vi "Demo_Main.vi"() -> ()   [LabVIEW 2011]
uses:
  ControlCAN/ControlCAN.llb/DevType.ctl
  ControlCAN/ControlCAN.llb/CAN Channel.ctl
  ControlCAN/ControlCAN.llb/InitFlag.ctl
  ControlCAN/ControlCAN.llb/Mode.ctl
  ControlCAN/ControlCAN.llb/Fliter.ctl
  ControlCAN/ControlCAN.llb/VCI_CAN_OBJ.ctl
  ControlCAN/ControlCAN.llb/VCI_INIT_CONFIG.ctl
  ControlCAN/ControlCAN.llb/Return Val.ctl
  ControlCAN/ControlCAN.lvlib
panel:
  in  "Clear":bool
  out "RecvCnt":u32 caption="接收统计"
  out "SendCnt":u32 caption="发送统计"
  in  "Format":u8(ring) items=["标准帧", "扩展帧"]
  in  "Type":u8(ring) items=["数据帧", "远程帧"]
  in  "Data":string="00 01 02 03 04 05 06 07"
  in  "ID":u32=291 format="0x%x"
  in  "list":i32(listbox)
  in  "Send":bool
  in  "RcvEnable":bool=TRUE
  out "Open":bool
  in  "Fliter":T1=1 items=["接收所有类型"=1, "只接收标准帧"=2, "只接收扩展帧"=3]
  in  "kBaudRate":u8(ring)=15 caption="波特率" items=["5k bps"=1, "10k bps"=2, "20k bps"=3, "40k bps"=4, "50k bps"=5, "80k bps"=6, "100k bps"=7, "125k bps"=8, "200k bps"=9, "250k bps"=10, "400k bps"=11, "500k bps"=12, "666k bps"=13, "800k bps"=14, "1000k bps"=15, "33.33k bps"=16, "66.66k bps"=17, "83.33k bps"=18]
  in  "Mode":T2=2 caption="工作模式" items=["正常工作", "仅侦听模式", "自测模式（环回）"]
  in  "InitFlag":T3=1 caption="保留值" items=["使用界面设置参数"=1]
  in  "AccMask":u32=4294967295 caption="接收屏蔽码" format="%08x"
  in  "AccCode":u32 caption="接收过滤码" format="%08x"
  in  "Close":bool
  in  "Open":bool
  in  "Channel":T4 caption="CAN通道" items=["通道1", "通道2"]
  in  "DevType":T5=4 caption="设备类型" items=["USB-CAN"=3, "USB-CAN2"=4]
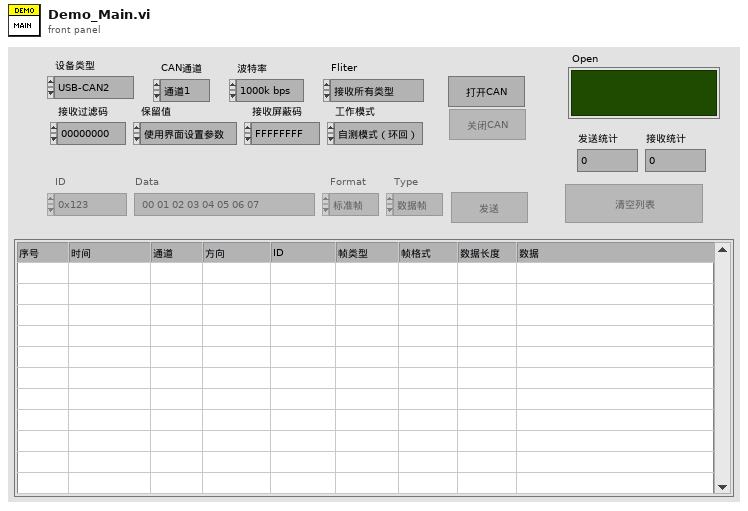
[diagram p1: front panel]
types:
  T1 = typedef "ControlCAN.lvlib/Fliter.ctl" = u8
  T2 = typedef "ControlCAN.lvlib/Mode.ctl" = u8
  T3 = typedef "ControlCAN.lvlib/InitFlag.ctl" = u32
  T4 = typedef "ControlCAN.lvlib/CAN Channel.ctl" = u32
  T5 = typedef "ControlCAN.lvlib/DevType.ctl" = u32
  T6 = typedef "ControlCAN.lvlib/VCI_CAN_OBJ.ctl" = cluster{"ID":u32, "TimeStamp":u32, "TimeFlag":u8, "SendType":u8, "RemoteFlag":u8, "ExternFlag":u8, "DataLen":u8, "Data":u8[], "Reserved":u8[]}
  T7 = cluster{"Type":enum16{"接收", "发送"}, "Channel":T4, "Time":timestamp, "VCI_CAN_OBJ":T6}[]
  T8 = cluster{"Type":enum16{"接收", "发送"}, "Channel":T4, "Time":timestamp, "VCI_CAN_OBJ":T6}
  T9 = typedef "ControlCAN.lvlib/VCI_INIT_CONFIG.ctl" = cluster{"AccCode":u32, "AccMask":u32, "InitFlag":T3, "Fliter":T1, "Timing0":u8, "Timing1":u8, "Mode":T2}
  T10 = cluster{"DevType":T5, "DevIndex":u32, "CanIndex":T4, "VCI_INIT_CONFIG":T9}
  T11 = typedef "ControlCAN.lvlib/Return Val.ctl" = i32
  T12 = enum32{"invalid app kind", "Development System", "Run Time System", "Student Edition", "Embedded LabVIEW", "Evaluation", "Custom"}
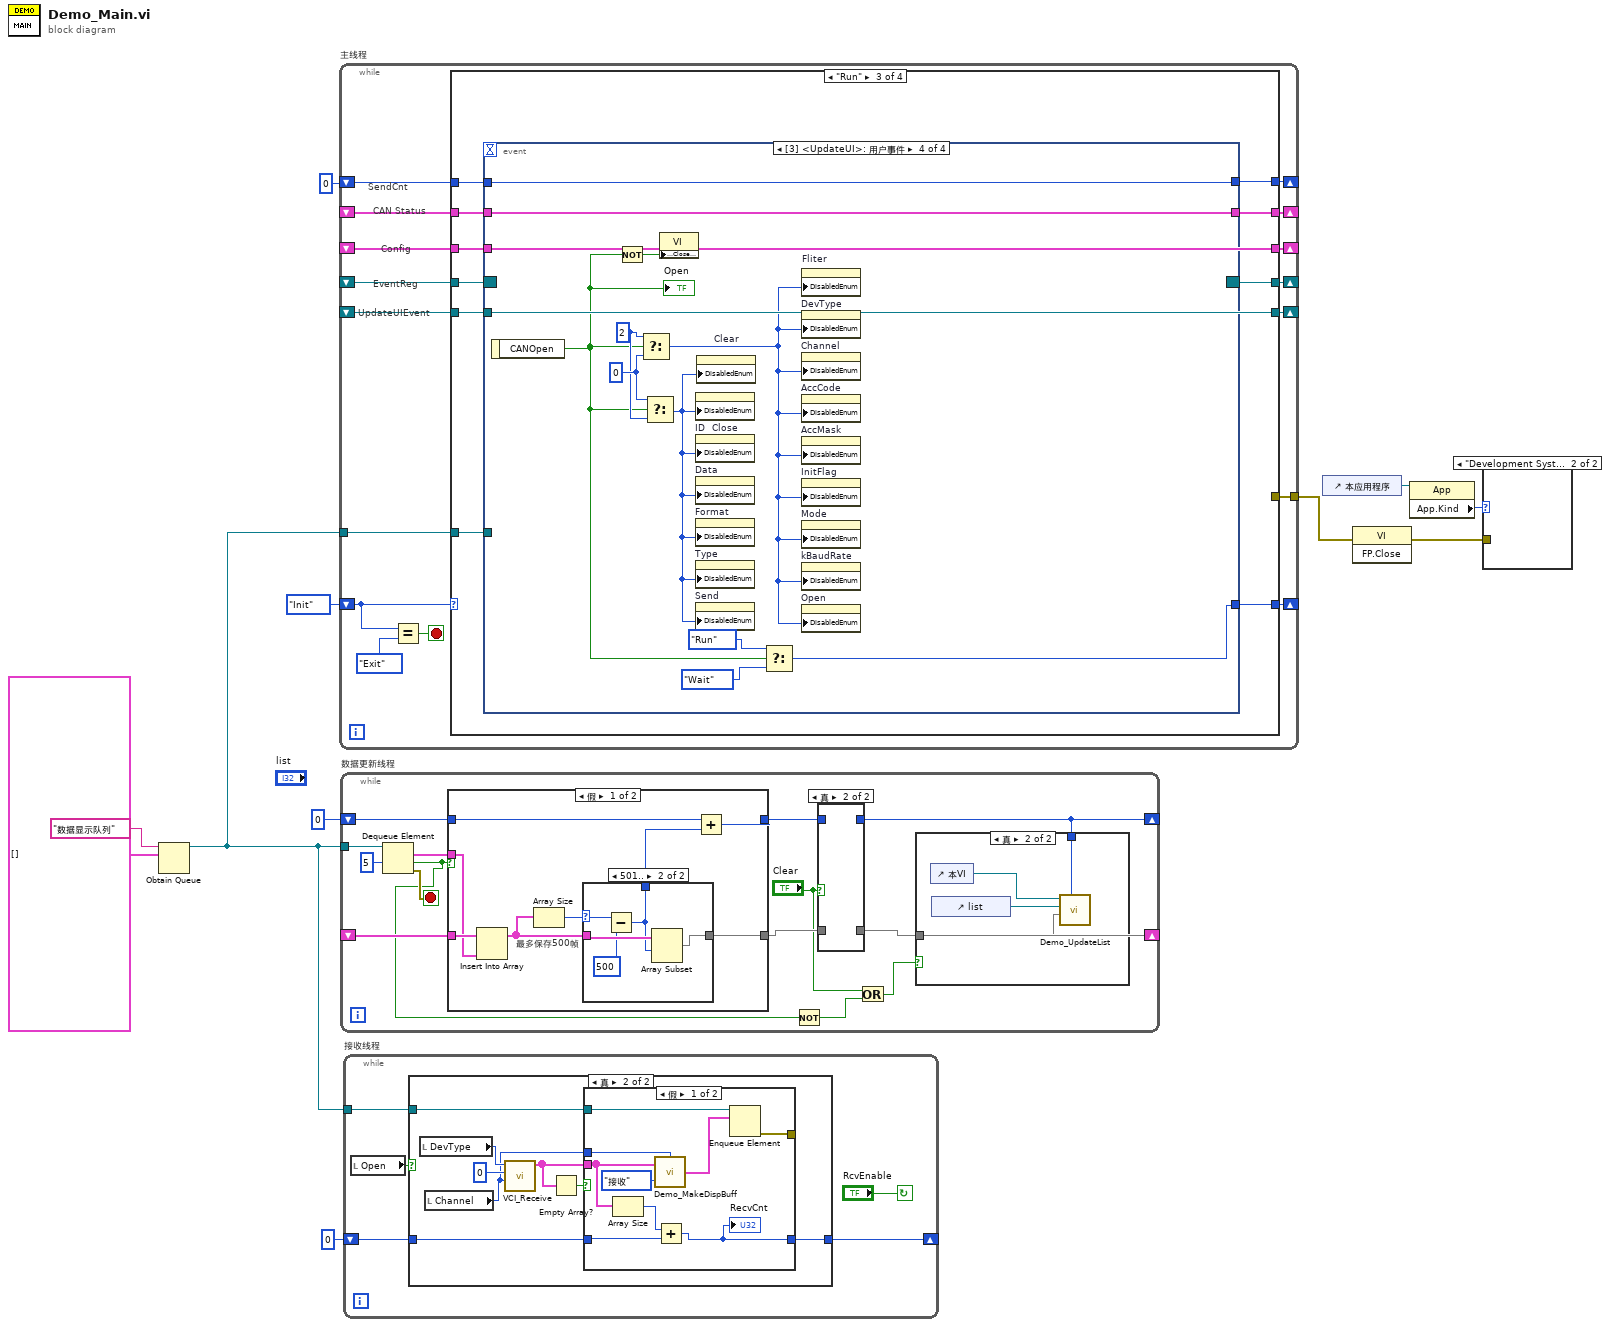
[diagram p0: block diagram]
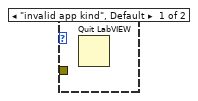
[diagram p2: hidden frame]
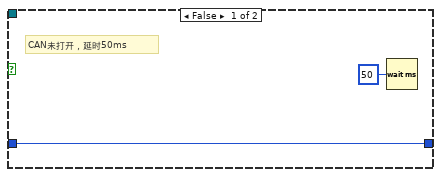
[diagram p7: hidden frame]
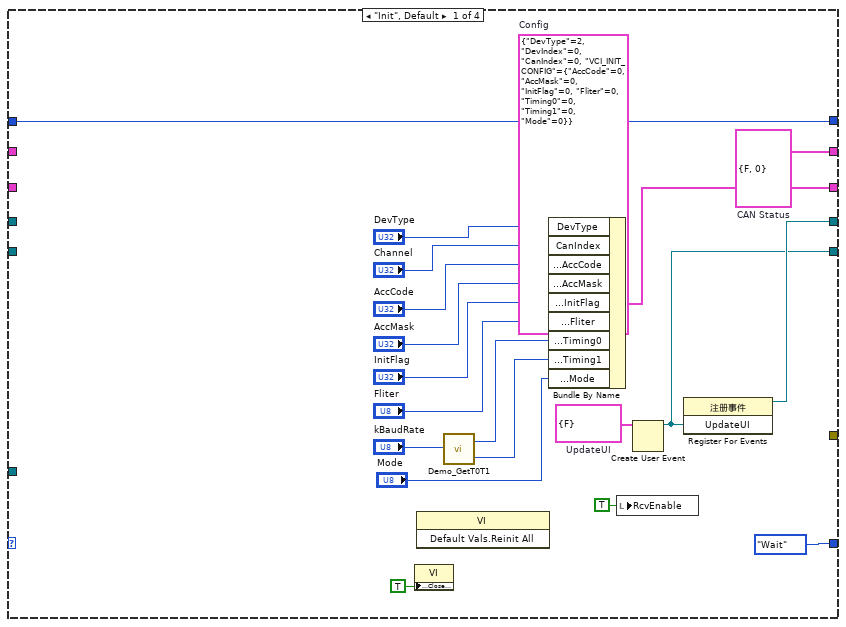
[diagram p9: hidden frame]
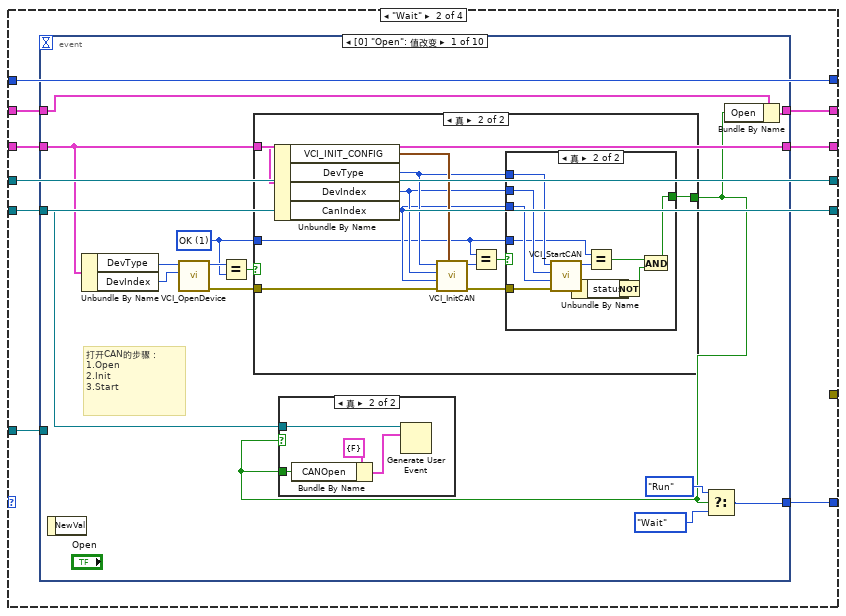
[diagram p10: hidden frame]
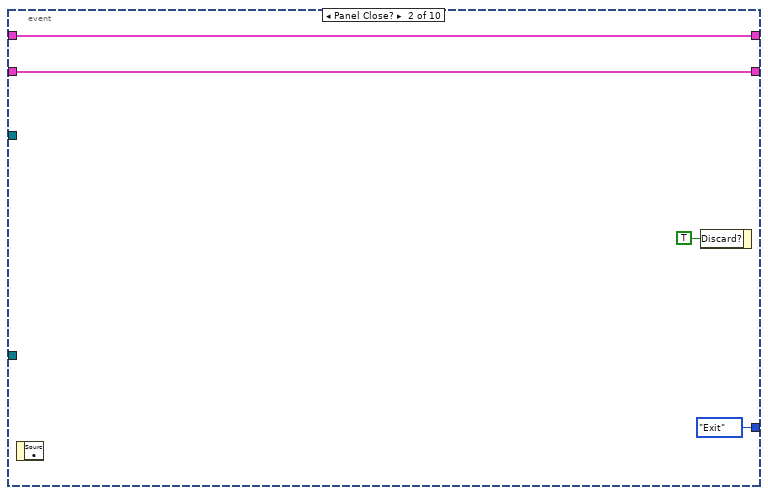
[diagram p14: hidden frame]
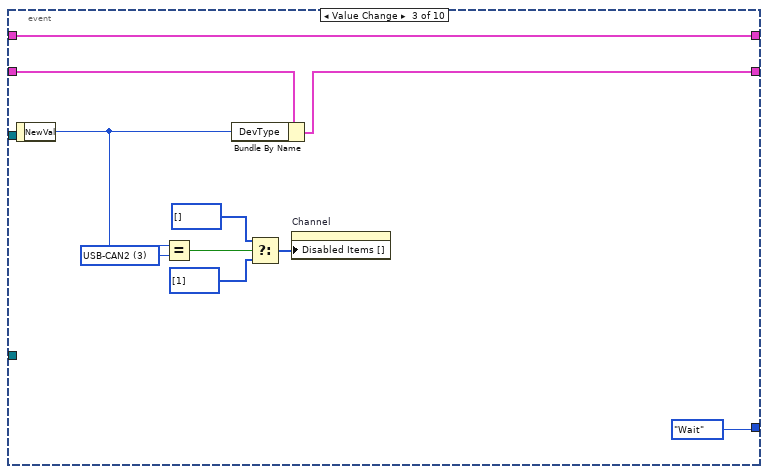
[diagram p15: hidden frame]
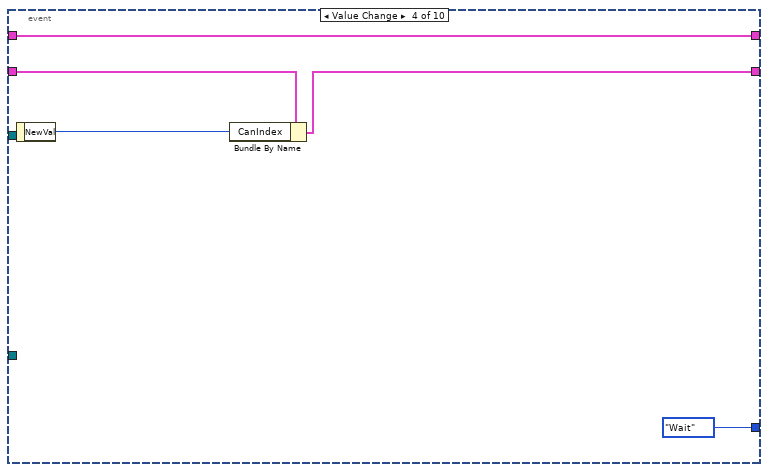
[diagram p16: hidden frame]
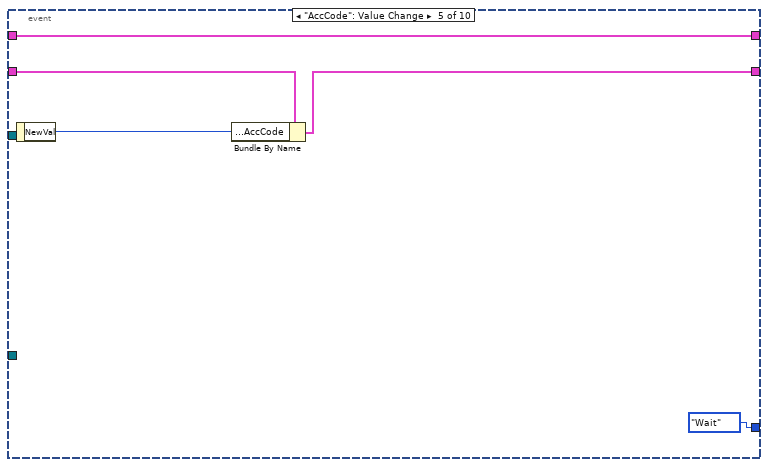
[diagram p17: hidden frame]
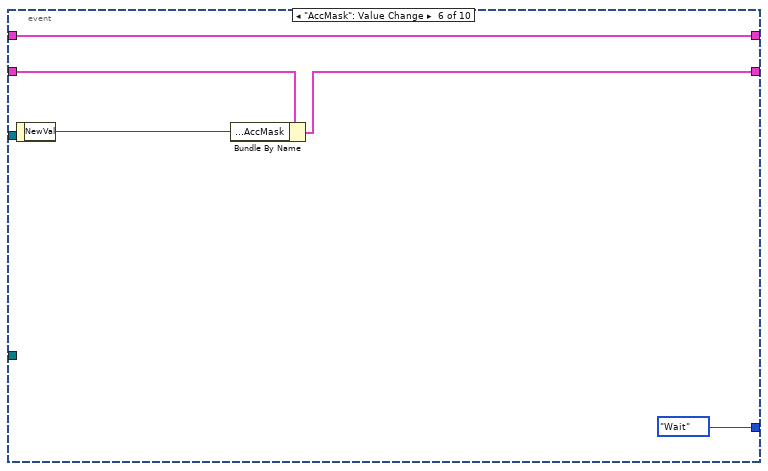
[diagram p18: hidden frame]
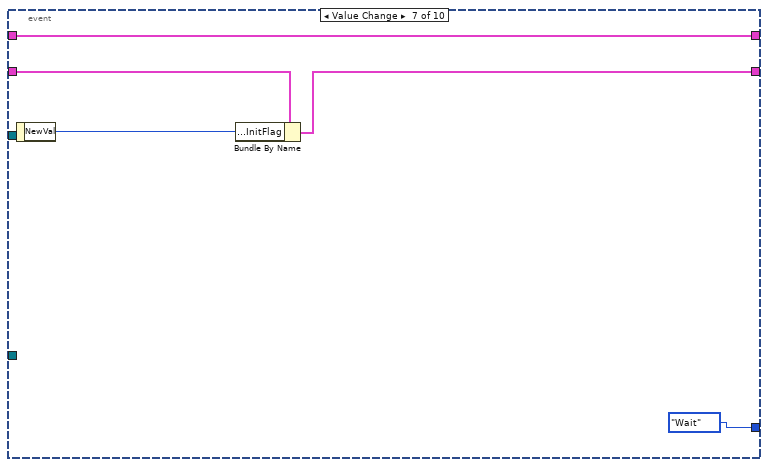
[diagram p19: hidden frame]
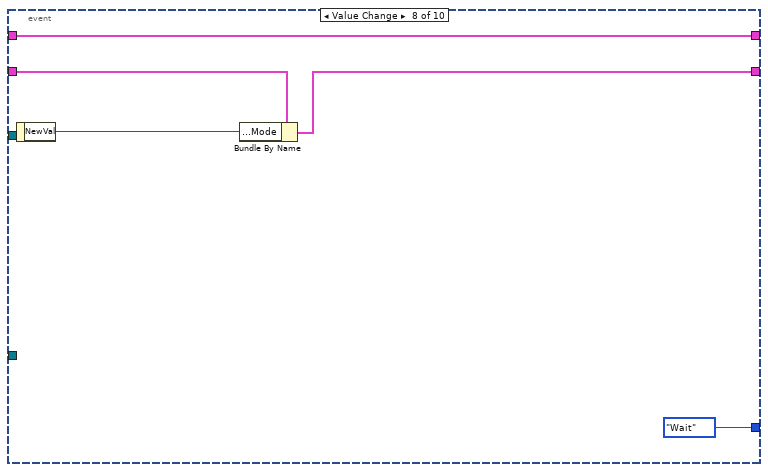
[diagram p20: hidden frame]
diagram:
  n1 = Obtain Queue(name (unnamed)="数据显示队列" ("名称（未命名）"), element data type=T7 []) -> (queue out=w8:refnum<queue>)  [unwired: 3 in, 2 out]
  n2 = while "主线程" {
    shift-right: [w23] -> _
    shift-left: enum16{"Init", "Wait", "Run", "Exit"}."Init" -> [w26]
    shift-right: [w24] -> _
    shift-left: _ -> [w25]
    shift-right: [w22] -> _
    shift-left: _ -> [w21]
    tunnel: w8 -> [w20]
    shift-right: [w18] -> _
    shift-left: _ -> [w17]
    shift-right: [w16] -> _
    shift-left: _ -> [w15]
    shift-right: [w13] -> _
    shift-left: u32 0 -> [w14]
    tunnel: [w12] -> w2
    stop <- w27 stop-if-true
    # "CAN Status"
    # "Config"
    # "EventReg"
    # "UpdateUIEvent"
    # "SendCnt"
    n3 = Equal?(x=w26, y=enum16{"Init", "Wait", "Run", "Exit"}."Exit") -> (x = y?=w27:bool)
    n4 = case shown="\"Run\"" w26 {
      tunnel: w25 -> [_ w56 w155 w214]
      tunnel: [w47 w55 w154 w214] -> w24
      tunnel: [enum16{"Init", "Wait", "Run", "Exit"}."Wait" w52 w157 enum16{"Init", "Wait", "Run", "Exit"}."Exit"] -> w23
      tunnel: [w43 w53 w153 w212] -> w22
      tunnel: w21 -> [_ w54 w153 w212]
      tunnel: w20 -> [_ w51 w156 w218]
      tunnel: [w35 w50 w151 w217] -> w18
      tunnel: w17 -> [_ w50 w152 w217]
      tunnel: [w34 w49 w150 w215] -> w16
      tunnel: w15 -> [_ w49 w150 w215]
      tunnel: w14 -> [w32 w48 w149 w210]
      tunnel: [w32 w48 w148 w210] -> w13
      tunnel: [_ _ _ errorcluster {"status"=FALSE, "code"=0, "source"=""} ("error constant")] -> w12
      frame "Init", Default {
        w36 = cluster{"CANOpen":bool} {"CANOpen"=FALSE}  # UpdateUI
        w46 = T10 {"DevType"=2, "DevIndex"=0, "CanIndex"=0, "VCI_INIT_CONFIG"={"AccCode"=0, "AccMask"=0, "InitFlag"=0, "Fliter"=0, "Timing0"=0, "Timing1"=0, "Mode"=0}}  # Config
        w47 = cluster{"Open":bool, "SendCnt":u32} {"Open"=FALSE, "SendCnt"=0}  # CAN Status
        n5 = property class="VI"("Front Panel.Closeable"=TRUE ("前面板窗口:可关闭")) -> ()  [unwired: 2 in, 2 out]
        n6 = invoke class="VI" method="Default Vals.Reinit All"() -> ()  [unwired: 3 in, 3 out]
        n7 = call "Demo_GetT0T1.vi"("kBaudRate"="kBaudRate") -> ("Timing0"=w29:u8, "Timing1"=w28:u8)
        n8 = Bundle By Name(cluster=w46, "DevType"="DevType", "CanIndex"="Channel", "VCI_INIT_CONFIG.AccCode"="AccCode", "VCI_INIT_CONFIG.AccMask"="AccMask", "VCI_INIT_CONFIG.InitFlag"="InitFlag", "VCI_INIT_CONFIG.Fliter"="Fliter", "VCI_INIT_CONFIG.Timing0"=w29, "VCI_INIT_CONFIG.Timing1"=w28, "VCI_INIT_CONFIG.Mode"="Mode") -> (w43:T10)
        n9 = local write "RcvEnable"(TRUE ("RcvEnable")) -> ()
        n10 = Create User Event(user event datatype=w36) -> (user event=w34:refnum<user-event>)  [unwired: 1 in, 1 out]
        n11 = register-events(w34) -> (reference out=w35:refnum<event-registration>)  [unwired: 2 in, 1 out]
      }
      frame "Wait" {
        n12 = event shown="[0] \"Open\": 值改变" {
          selector: _ -> [_ _ _ _ _ _ _ _ _ _]
          dyn-events: _ -> [_ _ _ _ _ _ _ _ _ _]
          timeout: _ -> [_ _ _ _ _ _ _ _ _ _]
          tunnel: w56 -> [w60 w100 w110 w115 w120 w125 w130 w135 w142 w147]
          tunnel: [w59 w100 w110 w115 w120 w125 w130 w135 w142 w147] -> w55
          tunnel: w54 -> [w70 w99 w109 w114 w119 w124 w129 w134 w141 w146]
          tunnel: [w70 w99 w108 w112 w117 w122 w127 w132 w140 w144] -> w53
          tunnel: [w61 enum16{"Init", "Wait", "Run", "Exit"}."Exit" enum16{"Init", "Wait", "Run", "Exit"}."Wait" enum16{"Init", "Wait", "Run", "Exit"}."Wait" enum16{"Init", "Wait", "Run", "Exit"}."Wait" enum16{"Init", "Wait", "Run", "Exit"}."Wait" enum16{"Init", "Wait", "Run", "Exit"}."Wait" enum16{"Init", "Wait", "Run", "Exit"}."Wait" enum16{"Init", "Wait", "Run", "Exit"}."Wait" enum16{"Init", "Wait", "Run", "Exit"}."Wait"] -> w52
          tunnel: w51 -> [_ _ _ _ _ _ _ _ _ _]
          tunnel: w49 -> [w58 _ _ _ _ _ _ _ _ _]
          event "Open": Value Change {
            w64 = T11 1 items=["OK"=1, "ERROR1"=0, "ERROR2"=-1] ("y")
            # "打开CAN的步骤：\n1.Open\n2.Init\n3.Start"
            n13 = event-data() -> ()  [unwired: 2 out]
            n14 = Unbundle By Name(w70) -> ("DevType"=w69:T5, "DevIndex"=w68:u32)
            n15 = call "VCI_OpenDevice.vi"("DevIndex"=w68, "DevType"=w69) -> ("error out"=w65:errorcluster, "Return Val"=w67:T11)  [unwired: 2 in, 6 out]
            n16 = Equal?(x=w67, y=w64) -> (x = y?=w66:bool)
            n17 = case shown="真" w66 {
              tunnel: w65 -> [_ w85]
              tunnel: w70 -> [_ w84]
              tunnel: w64 -> [_ w76]
              tunnel: [_ w75] -> w57
              frame False {
              }
              frame True {
                n18 = Unbundle By Name(w84) -> ("VCI_INIT_CONFIG"=w83:T9, "DevType"=w79:T5, "DevIndex"=w78:u32, "CanIndex"=w77:T4)
                n19 = call "VCI_InitCAN.vi"("VCI_INIT_CONFIG"=w83, "error in (no error)"=w85, "CANIndex"=w77, "DevIndex"=w78, "DevType"=w79) -> ("error out"=w80:errorcluster, "Return Val"=w82:T11)  [unwired: 5 out]
                n20 = Equal?(x=w76, y=w82) -> (x = y?=w81:bool)
                n21 = case shown="真" w81 {
                  tunnel: w80 -> [_ w96]
                  tunnel: w79 -> [_ w95]
                  tunnel: w78 -> [_ w94]
                  tunnel: w77 -> [_ w93]
                  tunnel: w76 -> [_ w91]
                  tunnel: [_ w87] -> w75
                  frame False {
                  }
                  frame True {
                    n22 = call "VCI_StartCAN.vi"("error in (no error)"=w96, "CANIndex"=w93, "DevIndex"=w94, "DevType"=w95) -> ("error out"=w89:errorcluster, "Return Val"=w92:T11)  [unwired: 6 out]
                    n23 = Unbundle By Name(w89) -> ("status"=w86:bool)
                    n24 = Equal?(x=w91, y=w92) -> (x = y?=w90:bool)
                    n25 = Not(x=w86) -> (.not. x?=w88:bool)
                    n26 = And(x=w90, y=w88) -> (x .and. y?=w87:bool)
                  }
                }
              }
            }
            n27 = case shown="真" w57 {
              tunnel: w58 -> [_ w74]
              tunnel: w57 -> [_ w72]
              frame False {
              }
              frame True {
                n28 = Bundle By Name(cluster=cluster{"CANOpen":bool} {"CANOpen"=FALSE} ("事件数据"), "CANOpen"=w72) -> (w71:cluster{"CANOpen":bool})
                n29 = Generate User Event(user event=w74, event data cluster=w71) -> ()  [unwired: 1 in, 2 out]
              }
            }
            n30 = Select(t=enum16{"Init", "Wait", "Run", "Exit"}."Run", s=w57, f=enum16{"Init", "Wait", "Run", "Exit"}."Wait") -> (s? t:f=w61:enum16{"Init", "Wait", "Run", "Exit"})
            n31 = Bundle By Name(cluster=w60, "Open"=w57) -> (w59:cluster{"Open":bool, "SendCnt":u32})
          }
          event Panel Close? {
            n32 = event-data() -> ()  [unwired: 2 out]
            n33 = event-data("Discard?"=TRUE ("放弃？")) -> ()  [unwired: 1 in, 1 out]
          }
          event Value Change {
            w106 = T5 3 items=["USB-CAN"=2, "USB-CAN2"=3] ("y")
            n34 = event-data() -> ("NewVal"=w107:T5)  [unwired: 1 out]
            n35 = Equal?(x=w107, y=w106) -> (x = y?=w105:bool)
            n36 = Bundle By Name(cluster=w109, "DevType"=w107) -> (w108:T10)
            n37 = Select(t=i32[] [] ("禁用项[]"), s=w105, f=i32[] [1] ("禁用项[]")) -> (s? t:f=w104:i32[])
            n38 = property on="Channel" class="Ring (严格)"("Disabled Items []"=w104) -> ()  [unwired: 2 in, 2 out]
          }
          event Value Change {
            n39 = event-data() -> ("NewVal"=w113:T4)  [unwired: 1 out]
            n40 = Bundle By Name(cluster=w114, "CanIndex"=w113) -> (w112:T10)
          }
          event "AccCode": Value Change {
            n41 = event-data() -> ("NewVal"=w118:u32)  [unwired: 1 out]
            n42 = Bundle By Name(cluster=w119, "VCI_INIT_CONFIG.AccCode"=w118) -> (w117:T10)
          }
          event "AccMask": Value Change {
            n43 = event-data() -> ("NewVal"=w123:u32)  [unwired: 1 out]
            n44 = Bundle By Name(cluster=w124, "VCI_INIT_CONFIG.AccMask"=w123) -> (w122:T10)
          }
          event Value Change {
            n45 = event-data() -> ("NewVal"=w128:T3)  [unwired: 1 out]
            n46 = Bundle By Name(cluster=w129, "VCI_INIT_CONFIG.InitFlag"=w128) -> (w127:T10)
          }
          event Value Change {
            n47 = event-data() -> ("NewVal"=w133:T2)  [unwired: 1 out]
            n48 = Bundle By Name(cluster=w134, "VCI_INIT_CONFIG.Mode"=w133) -> (w132:T10)
          }
          event "kBaudRate": Value Change {
            n49 = event-data() -> ("NewVal"=w138:u8)  [unwired: 1 out]
            n50 = call "Demo_GetT0T1.vi"("kBaudRate"=w138) -> ("Timing0"=w137:u8, "Timing1"=w136:u8)
            n51 = Bundle By Name(cluster=w141, "VCI_INIT_CONFIG.Timing0"=w137, "VCI_INIT_CONFIG.Timing1"=w136) -> (w140:T10)
          }
          event Value Change {
            n52 = event-data() -> ("NewVal"=w145:T1)  [unwired: 1 out]
            n53 = Bundle By Name(cluster=w146, "VCI_INIT_CONFIG.Fliter"=w145) -> (w144:T10)
          }
        }
      }
      frame "Run" {
        n54 = event shown="[3] <UpdateUI>: 用户事件" {
          selector: w152 -> [_ _ _ _]
          dyn-events: [_ _ _ _] -> w151
          timeout: _ -> [_ _ _ _]
          tunnel: [enum16{"Init", "Wait", "Run", "Exit"}."Run" enum16{"Init", "Wait", "Run", "Exit"}."Run" enum16{"Init", "Wait", "Run", "Exit"}."Run" w202] -> w157
          tunnel: w156 -> [_ w171 _ _]
          tunnel: [w159 w182 w189 w208] -> w154
          tunnel: w155 -> [w159 w182 w191 w208]
          tunnel: w153 -> [_ w177 w196 _]
          tunnel: w150 -> [_ _ w188 _]
          tunnel: w149 -> [w158 w166 w184 w201]
          tunnel: [w158 w165 w184 w201] -> w148
          event Timeout {
            n55 = event-data() -> ()  [unwired: 3 out]
          }
          event "Send": Value Change {
            n56 = event-data() -> ()  [unwired: 2 out]
            n57 = Increment(x=w166) -> (x+1=w165:u32)
            "SendCnt" <- w165
            n58 = call "Demo_MakeData.vi"("DataString"="Data") -> ("Data"=w172:u8[], "DataLen"=w173:u8)  [unwired: 9 out]
            n59 = Bundle By Name(cluster=T6 {"ID"=0, "TimeStamp"=0, "TimeFlag"=0, "SendType"=0, "RemoteFlag"=0, "ExternFlag"=0, "DataLen"=0, "Data"=[], "Reserved"=[]} ("Send"), "ID"="ID", "RemoteFlag"="Type", "ExternFlag"="Format", "DataLen"=w173, "Data"=w172) -> (w163:T6)
            n60 = Build Array(w163) -> (w164:T6[])
            n61 = Get Date/Time In Seconds() -> (seconds since 1Jan1904=w167:timestamp)
            n62 = Unbundle By Name(w177) -> ("DevType"=w176:T5, "DevIndex"=w175:u32, "CanIndex"=w168:T4)
            n63 = Bundle By Name(cluster=T8 {"Type"=enum."发送", "Channel"=0, "Time"=timestamp(0 s since 1904-01-01), "VCI_CAN_OBJ"={"ID"=0, "TimeStamp"=0, "TimeFlag"=0, "SendType"=0, "RemoteFlag"=0, "ExternFlag"=0, "DataLen"=0, "Data"=[], "Reserved"=[]}}, "Type"=enum16{"接收", "发送"}."发送", "Channel"=w168, "Time"=w167, "VCI_CAN_OBJ"=w163) -> (w162:T8)
            n64 = call "VCI_Transmit.vi"("Buffer"=w164, "CANIndex"=w168, "DevIndex"=w175, "DevType"=w176) -> ()  [unwired: 1 in, 7 out]
            n65 = Build Array(w162) -> (w161:T7)
            n66 = Enqueue Element(queue=w171, element=w161) -> ()  [unwired: 1 in, 4 out]
          }
          event "Close": Value Change {
            w192 = T11 1 items=["OK"=1, "ERROR1"=0, "ERROR2"=-1] ("y")
            n67 = event-data() -> ()  [unwired: 2 out]
            n68 = Unbundle By Name(w196) -> ("DevType"=w195:T5, "DevIndex"=w194:u32)
            n69 = call "VCI_CloseDevice.vi"("DevIndex"=w194, "DevType"=w195) -> ("Return Val"=w193:T11)  [unwired: 1 in, 8 out]
            n70 = Equal?(x=w193, y=w192) -> (x = y?=w190:bool)
            n71 = Not(x=w190) -> (.not. x?=w186:bool)
            n72 = Bundle By Name(cluster=cluster{"CANOpen":bool} {"CANOpen"=FALSE} ("事件数据"), "CANOpen"=w186) -> (w185:cluster{"CANOpen":bool})
            n73 = Bundle By Name(cluster=w191, "Open"=w186) -> (w189:cluster{"Open":bool, "SendCnt":u32})
            n74 = local write "Open"(w186) -> ()
            n75 = Generate User Event(user event=w188, event data cluster=w185) -> ()  [unwired: 1 in, 2 out]
          }
          event User Event {
            w206 = 0
            w205 = 2
            n76 = event-data() -> ("CANOpen"=w198:bool)  [unwired: 1 out]
            "Open" <- w198
            n77 = Not(x=w198) -> (.not. x?=w199:bool)
            n78 = Select(t=w205, s=w198, f=w206) -> (s? t:f=w207:i32)
            n79 = Select(t=w206, s=w198, f=w205) -> (s? t:f=w200:i32)
            n80 = property class="VI"("Front Panel.Closeable"=w199) -> ()  [unwired: 2 in, 2 out]
            n81 = property on="Close" class="Bool"("DisabledEnum"=w200) -> ()  [unwired: 2 in, 2 out]
            n82 = property on="ID" class="DigNum (严格)"("DisabledEnum"=w200) -> ()  [unwired: 2 in, 2 out]
            n83 = property on="Data" class="Str"("DisabledEnum"=w200) -> ()  [unwired: 2 in, 2 out]
            n84 = property on="Format" class="Ring (严格)"("DisabledEnum"=w200) -> ()  [unwired: 2 in, 2 out]
            n85 = property on="Type" class="Ring (严格)"("DisabledEnum"=w200) -> ()  [unwired: 2 in, 2 out]
            n86 = property on="Send" class="Bool"("DisabledEnum"=w200) -> ()  [unwired: 2 in, 2 out]
            n87 = property on="Clear" class="Bool"("DisabledEnum"=w200) -> ()  [unwired: 2 in, 2 out]
            n88 = Select(t=enum16{"Init", "Wait", "Run", "Exit"}."Run", s=w198, f=enum16{"Init", "Wait", "Run", "Exit"}."Wait") -> (s? t:f=w202:enum16{"Init", "Wait", "Run", "Exit"})
            n89 = property on="Fliter" class="Ring (严格)"("DisabledEnum"=w207) -> ()  [unwired: 2 in, 2 out]
            n90 = property on="DevType" class="Ring (严格)"("DisabledEnum"=w207) -> ()  [unwired: 2 in, 2 out]
            n91 = property on="Channel" class="Ring (严格)"("DisabledEnum"=w207) -> ()  [unwired: 2 in, 2 out]
            n92 = property on="AccCode" class="DigNum (严格)"("DisabledEnum"=w207) -> ()  [unwired: 2 in, 2 out]
            n93 = property on="AccMask" class="DigNum (严格)"("DisabledEnum"=w207) -> ()  [unwired: 2 in, 2 out]
            n94 = property on="InitFlag" class="Ring (严格)"("DisabledEnum"=w207) -> ()  [unwired: 2 in, 2 out]
            n95 = property on="Mode" class="Ring (严格)"("DisabledEnum"=w207) -> ()  [unwired: 2 in, 2 out]
            n96 = property on="kBaudRate" class="Ring (严格)"("DisabledEnum"=w207) -> ()  [unwired: 2 in, 2 out]
            n97 = property on="Open" class="Bool"("DisabledEnum"=w207) -> ()  [unwired: 2 in, 2 out]
          }
        }
      }
      frame "Exit" {
        n98 = Release Queue(queue=w218) -> ()  [unwired: 1 in, 4 out]
        n99 = Unregister For Events(event registration refnum=w217) -> (error out=w216:errorcluster)  [unwired: 1 in]
        n100 = Destroy User Event(user event=w215, error in=w216) -> ()  [unwired: 1 out]
        n101 = Unbundle By Name(w214) -> ("Open"=w213:bool)
        n102 = case shown="真" w213 {
          tunnel: w212 -> [_ w222]
          frame False {
          }
          frame True {
            n103 = Unbundle By Name(w222) -> ("DevType"=w221:T5, "DevIndex"=w220:u32)
            n104 = call "VCI_CloseDevice.vi"("DevIndex"=w220, "DevType"=w221) -> ()  [unwired: 1 in, 9 out]
          }
        }
        n105 = local write "RcvEnable"(FALSE ("RcvEnable")) -> ()
      }
    }
  }
  n106 = while "数据更新线程" {
    tunnel: w8 -> [w236]
    shift-right: [w227] -> _
    shift-left: _ -> [w232]
    shift-right: [w228] -> _
    shift-left: 0 -> [w231]
    stop <- w234 stop-if-true
    n107 = Dequeue Element(queue=w236, timeout in ms (-1)=5 ("超时毫秒(-1)")) -> (element=w233:T7, timed out?=w226:bool, error out=w234:errorcluster)  [unwired: 1 in, 1 out]
    n108 = case shown="假" w226 {
      tunnel: w233 -> [w247 _]
      tunnel: w232 -> [w250 w258]
      tunnel: [w243 w258] -> w230
      tunnel: w231 -> [w246 w257]
      tunnel: [w244 w257] -> w229
      frame False {
        n109 = Insert Into Array(array=w250, new element=w247) -> (w248:T7)  [unwired: 1 in]
        n110 = Array Size(array=w248) -> (size(s)=w249:i32)
        n111 = case "最多保存500帧" shown="501.." w249 {
          selector: w249 -> [_ w255]
          tunnel: w248 -> [w251 w256]
          tunnel: [w251 w253] -> w243
          tunnel: [_ w252] -> w245
          frame 0, Default {
          }
          frame 501.. {
            n112 = Subtract(x=w255, y=500) -> (x-y=w252:i32)
            n113 = Array Subset(array=w256, index=w252) -> (w253:T7)  [unwired: 1 in]
          }
        }
        n114 = Add(x=w246, y=w245) -> (x+y=w244:i32)
      }
      frame True {
      }
    }
    n115 = Not(x=w226) -> (.not. x?=w225:bool)
    n116 = case shown="真" "Clear" {
      tunnel: w229 -> [w241 _]
      tunnel: w230 -> [w242 _]
      tunnel: [w242 _] -> w227
      tunnel: [w241 _] -> w228
      frame False {
      }
      frame True {
      }
    }
    n117 = Or(x="Clear", y=w225) -> (x .or. y?=w224:bool)
    n118 = case shown="真" w224 {
      tunnel: w228 -> [_ w238]
      tunnel: w227 -> [_ w237]
      frame False {
      }
      frame True {
        n119 = control-ref of="本VI"() -> (w239:refnum<vi>)
        n120 = control-ref of="list"() -> (w240:refnum<vi>)
        n121 = call "Demo_UpdateList.vi"("Offset"=w238, "Buffer"=w237, "list"=w240, "MainVi"=w239) -> ()  [unwired: 8 out]
      }
    }
  }
  n122 = while "接收线程" {
    tunnel: w8 -> [w261]
    shift-right: [w259] -> _
    shift-left: u32 0 ("RecvCnt") -> [w260]
    stop <- "RcvEnable" continue-if-true
    n123 = local read "Open"() -> (w262:bool)
    n124 = case shown="真" w262 {
      tunnel: w261 -> [_ w269]
      tunnel: w260 -> [w264 w268]
      tunnel: [w264 w267] -> w259
      frame False {
        # "CAN未打开，延时50ms"
        n125 = Wait (ms)(milliseconds to wait=u32 50 ("等待时间（毫秒）")) -> ()  [unwired: 1 out]
      }
      frame True {
        n126 = local read "DevType"() -> (w273:T5)
        n127 = local read "Channel"() -> (w266:T4)
        n128 = call "VCI_Receive.vi"("CANIndex"=w266, "DevIndex"=u32 0, "DevType"=w273) -> ("Recieve"=w270:T6[])  [unwired: 3 in, 5 out]
        n129 = Empty Array?(array=w270) -> (empty?=w271:bool)
        n130 = case shown="假" w271 {
          tunnel: w269 -> [w282 _]
          tunnel: w270 -> [w278 _]
          tunnel: [w279 _] -> _
          tunnel: w268 -> [w276 w283]
          tunnel: [w275 w283] -> w267
          tunnel: w266 -> [w274 _]
          frame False {
            n131 = Array Size(array=w278) -> (size(s)=w277:i32)
            n132 = call "Demo_MakeDispBuff.vi"("Channel"=w274, "Type"=enum16{"接收", "发送"}."接收", "OBJs"=w278) -> ("Buffer"=w280:T7)
            n133 = Add(x=w277, y=w276) -> (x+y=w275:u32)
            "RecvCnt" <- w275
            n134 = Enqueue Element(queue=w282, element=w280) -> (error out=w279:errorcluster)  [unwired: 1 in, 3 out]
          }
          frame True {
          }
        }
      }
    }
  }
  n135 = control-ref of="本应用程序"() -> (w4:refnum<vi>)
  n136 = invoke class="VI" method="FP.Close"(error in=w2) -> (error out=w1:errorcluster)  [unwired: 2 in, 2 out]
  n137 = property class="App"(reference=w4) -> ("App.Kind"=w3:T12)  [unwired: 1 in, 2 out]
  n138 = case shown="\"Development System\"" w3 {
    tunnel: w1 -> [_ _]
    frame "invalid app kind", Default {
      n139 = Quit LabVIEW() -> ()  [unwired: 1 out]
    }
    frame "Development System" {
    }
  }
